vi "meas_Ia.vi"(8 "error in (no error)":errorcluster, 11 "3_amp_volt in":refnum<class "3_amp_volt.lvclass">) -> (0 "error out":errorcluster, 2 "Measured Ia":sgl, 3 "3_amp_volt out":refnum<class "3_amp_volt.lvclass">)   [LabVIEW 2018, in "3_amp_volt.lvclass"]
uses:
  3_amp_volt.lvclass
  3_amp_volt.lvclass/3_amp_volt.ctl
  <vilib>/Plasmionique/MB Master/MB_Master_Serial/MB_Master_Serial.lvclass
  C:/Program Files/National Instruments/LabVIEW 2018/vi.lib/Plasmionique/MB Master/MB_Master/MB_Master.lvclass
  <vilib>/Plasmionique/MB Master/MB Master.lvlib
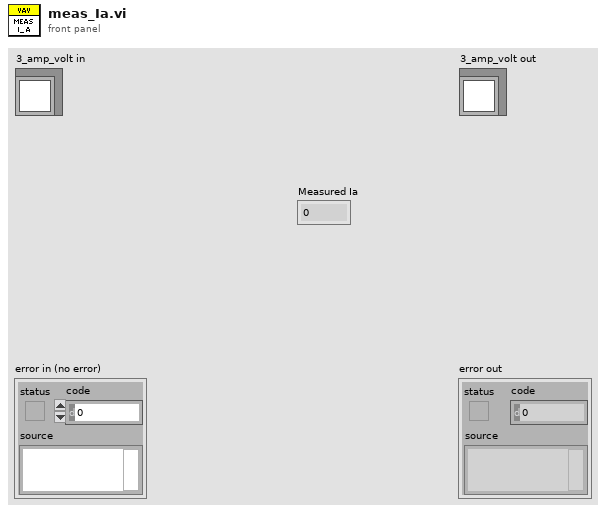
[diagram p1: front panel]
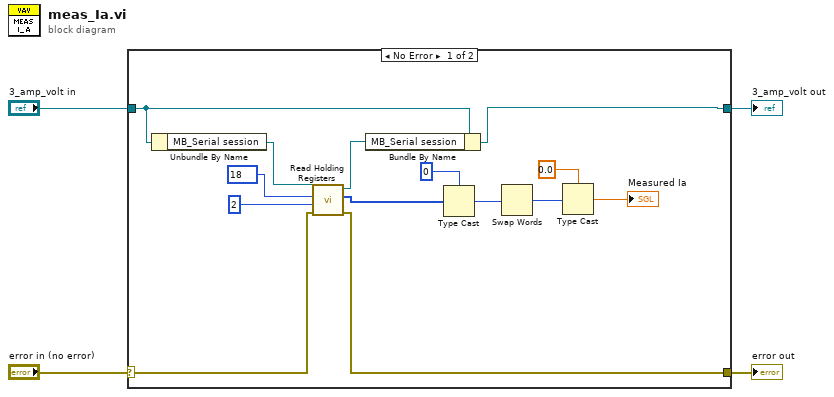
[diagram p0: block diagram]
diagram:
  n1 = case shown="No Error" "error in (no error)" {
    selector: "error in (no error)" -> [w6 w20]
    tunnel: [w5 w20] -> w3
    tunnel: [w7 w19] -> w1
    tunnel: "3_amp_volt in" -> [w8 w19]
    frame No Error {
      n2 = Unbundle By Name(w8) -> ("MB_Serial session"=w18:refnum<class "MB_Master_Serial.lvclass">)
      n3 = call <vilib>:"Read Holding Registers.vi"("error in (no error)"=w6, "quantity"=u16 2, "starting address"=u16 18, "MB session in"=w18) -> ("error out"=w5:errorcluster, "Registers"=w14:u16[], "MB session out"=w15:refnum<class "MB_Master_Serial.lvclass">)  [unwired: 5 in]
      n4 = Bundle By Name(cluster=w8, "MB_Serial session"=w15) -> (w7:refnum<class "3_amp_volt.lvclass">)
      n5 = Type Cast(type=u32 0 ("quantity"), x=w14) -> (*(type *) &x=w12:u32)
      n6 = Swap Words(1:w12) -> (0:w11:u32)
      n7 = Type Cast(type=sgl 0.0 ("quantity"), x=w11) -> (*(type *) &x=→"Measured Ia":sgl)
    }
    frame Error {
    }
  }
  "error out" <- w3
  "3_amp_volt out" <- w1
